vi "Temperature Monitor.vi"() -> ()   [LabVIEW 2012]
doc: "This VI is the solution to an exercise in the LabVIEW Core 1 course.\n\nIt uses a While Loop and shift registers to average data. No hardware is necessary."
panel:
  in  "Stop Button":bool
  out "Temperature History":dbl(graph)
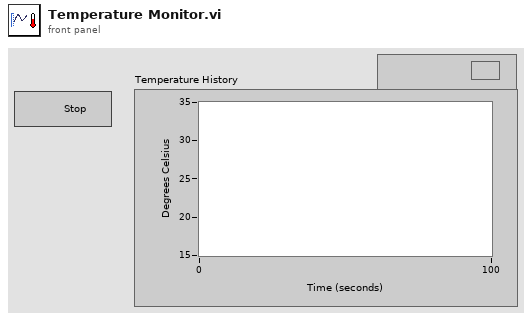
[diagram p1: front panel]
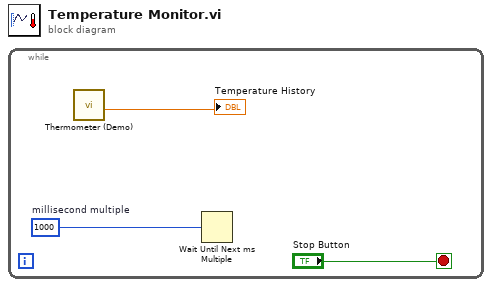
[diagram p0: block diagram]
diagram:
  n1 = while {
    stop <- "Stop Button" stop-if-true
    w3 = u32 1000  # millisecond multiple
    n2 = call "Thermometer (Demo).vi"() -> ("Temperature Value"=→"Temperature History":dbl)  [unwired: 11 in]
    n3 = Wait Until Next ms Multiple(millisecond multiple=w3) -> ()  [unwired: 1 out]
  }
